vi "set Parameters.vi"(8 "error in (no error)":errorcluster, 11 "EMTestCWS500N in":refnum<class "EMTestCWS500N.lvclass">) -> (0 "error out":errorcluster, 2 "Parameters":u32[](array[numeric]), 3 "EMTestCWS500N out":refnum<class "EMTestCWS500N.lvclass">)   [LabVIEW 2013, in "EMTestCWS500N.lvclass"]
uses:
  EMTestCWS500N.lvclass
panel:
  in  "Leerlaufspannung rms unmoduliert":u32
  in  "Dwell Time (s)":dbl
  in  "Start Frequency (khz)":u32
  in  "End Frequency (khz)":u32
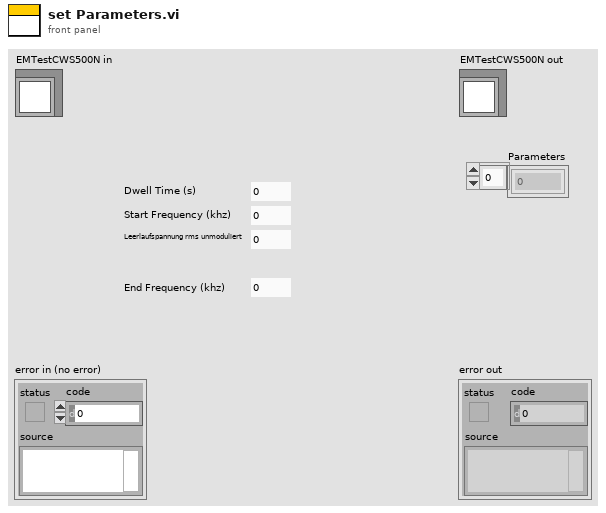
[diagram p1: front panel]
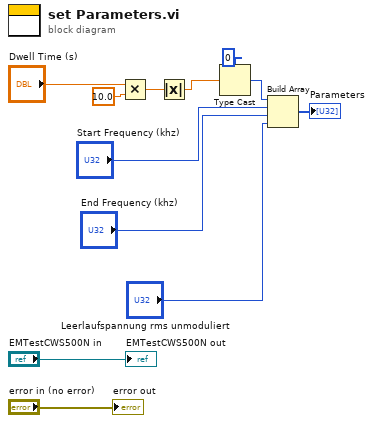
[diagram p0: block diagram]
diagram:
  n1 = Multiply(x="Dwell Time (s)", y=10.0) -> (x*y=w9:dbl)
  n2 = Absolute Value(x=w9) -> (abs(x)=w2:dbl)
  n3 = Type Cast(type=u32 0 ("unit (none)"), x=w2) -> (*(type *) &x=w1:u32)
  n4 = Build Array(w1, "Start Frequency (khz)", "End Frequency (khz)", "Leerlaufspannung rms unmoduliert") -> (→"Parameters":u32[])
  "error out" <- "error in (no error)"
  "EMTestCWS500N out" <- "EMTestCWS500N in"
